vi "GetImage.vi"(8 "error in (no error)":errorcluster, 11 "SVimage in":refnum<class "SVimage.lvclass">) -> (0 "error out":errorcluster, 1 "Image received":bool, 2 "Image Out":T1, 3 "SVimage out":refnum<class "SVimage.lvclass">)   [LabVIEW 2020, in "SVimage.lvclass"]
uses:
  SVimage.lvclass
  <vilib>/vision/Image Controls.llb/IMAQ Image.ctl
  SVimage.lvclass/SVimage.ctl
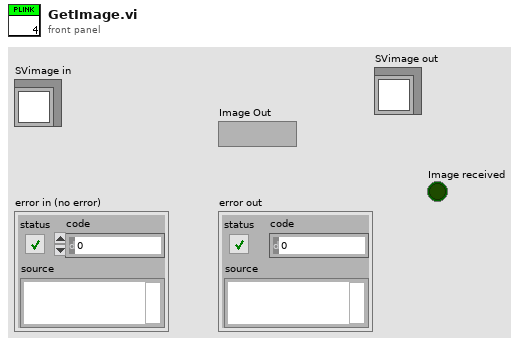
[diagram p1: front panel]
types:
  T1 = typedef "IMAQ Image.ctl" = refnum<image>
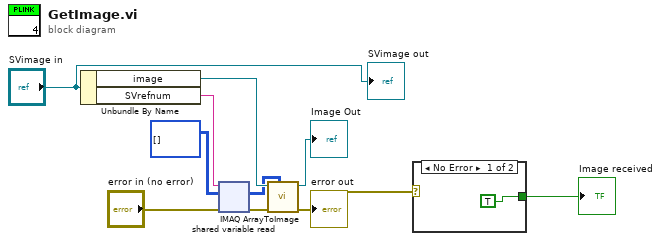
[diagram p0: block diagram]
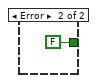
[diagram p2: hidden frame]
diagram:
  n1 = Unbundle By Name("SVimage in") -> ("image"=w8:T1, "SVrefnum"=w5:string)
  n2 = shared-variable-read(w5, "error in (no error)", u8[][] []) -> (w10:errorcluster, w7:u8[][])  [unwired: 2 out]
  n3 = call "IMAQ ArrayToImage"("Image Pixels (U16)"=w7, "error in (no error)"=w10, "Image"=w8) -> ("error out"=w2:errorcluster, "Image Out"=→"Image Out":T1)  [unwired: 7 in]
  "error out" <- w2
  n4 = case shown="No Error" w2 {
    tunnel: [TRUE ("Image received") FALSE ("Image received")] -> w1
    frame No Error {
    }
    frame Error {
    }
  }
  "Image received" <- w1
  "SVimage out" <- "SVimage in"
